vi "get_type_enum.vi"(11 "TypeDescriptor":refnum<class "TD.lvclass">) -> (2 "type":T1 format="%.0x", 3 "TypeDescriptor out":refnum<class "TD.lvclass">)   [LabVIEW 2020, in "variant.lvlib" / "type.lvlib" / "TD.lvclass"]
uses:
  TD.lvclass
  C:/projects/OpenG-Variant-Data-Library/source/library/Bytes/Bytes.lvclass
  Type Descriptor Enumeration.ctl
  TD.lvclass/TD.ctl
  Bytes/Bytes.lvclass/Bytes.ctl
  Bytes/from_byte_array.vi
  Bytes/Bytes.lvclass
  openg_variant.lvlib
  C:/projects/OpenG-Variant-Data-Library/source/library/LVData/Type Descriptor/TD.lvclass
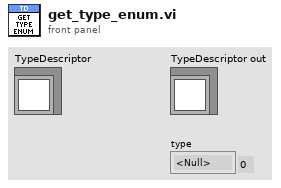
[diagram p1: front panel]
types:
  T1 = typedef "openg_variant.lvlib/Type Descriptor Enumeration.ctl" = enum8{"<Null>", "I8", "I16", "I32", "I64", "U8", "U16", "U32", "U64", "SGL", "DBL", "EXT", "CSG", "CDB", "CXT", "0x0F", "0x10", "0x11", "0x12", "0x13", "0x14", "Enum U8", "Enum U16", "Enum U32", "Enum U64", "SGL PQ", "DBL PQ", "EXT PQ", "CSG PQ", "CDB PQ", "CXT PQ", "0x1F", "0x20", "Boolean", "0x22", "0x23", "0x24", "0x25", "0x26", "0x27", "0x28", "0x29", "0x2A", "0x2B", "0x2C", "0x2D", "0x2E", "0x2F", "String", "0x31", "Path", "Pict", "0x34", "0x35", "0x36", "DAQ", "0x38", "0x39", "0x3A", "0x3B", "0x3C", "0x3D", "0x3E", "0x3F", "Array", "0x41", "0x42", "0x43", "0x44", "0x45", "0x46", "0x47", "0x48", "0x49", "0x4A", "0x4B", "0x4C", "0x4D", "0x4E", "0x4F", "Cluster", "0x51", "0x52", "Variant", "Waveform", "0x55", "0x56", "0x57", "0x58", "0x59", "0x5A", "0x5B", "0x5C", "0x5D", "0x5E", "Fixed Point", "0x60", "0x61", "0x62", "0x63", "0x64", "0x65", "0x66", "0x67", "0x68", "0x69", "0x6A", "0x6B", "0x6C", "0x6D", "0x6E", "0x6F", "Refnum", "0x71", "0x72", "Set Collection", "Map Collection"}
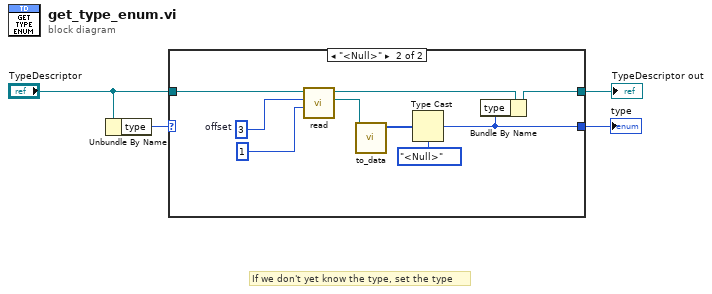
[diagram p0: block diagram]
diagram:
  # "If we don't yet know the type, set the type"
  n1 = Unbundle By Name("TypeDescriptor") -> ("type"=w1:T1)
  n2 = case shown="\"<Null>\"" w1 {
    selector: w1 -> [w5 _]
    tunnel: [w6 w9] -> w4
    tunnel: [w5 w8] -> w3
    tunnel: "TypeDescriptor" -> [w6 w7]
    frame Default {
    }
    frame "<Null>" {
      w14 = 3  # offset
      n3 = call "read.vi"("length (-1: rest)"=1, "offset (-1: current position)"=w14, "Bytes in"=w7) -> ("type to read"=w12:refnum<class "Bytes.lvclass">, "Bytes in"=w15:refnum<class "TD.lvclass">)  [unwired: 7 in]
      n4 = call "to_data.vi"("Bytes in"=w12) -> ("byte array"=w11:u8[])  [unwired: 10 in]
      n5 = Type Cast(type=Type_Descriptor_Enumeration."<Null>", x=w11) -> (*(type *) &x=w8:T1)
      n6 = Bundle By Name(cluster=w15, "type"=w8) -> (w9:refnum<class "TD.lvclass">)
    }
  }
  "TypeDescriptor out" <- w4
  "type" <- w3
